vi "Disabled - Load Constants (SubVI).vi"(9 "Robot Path":string="/c/tmp/auton/", 11 "Force Reload":bool) -> (0 "Constants Numeric\nArray":dbl[](array[numeric]), 1 "error out":errorcluster, 3 "Constants Header\nArray":string[](array[string]))   [LabVIEW 2019]
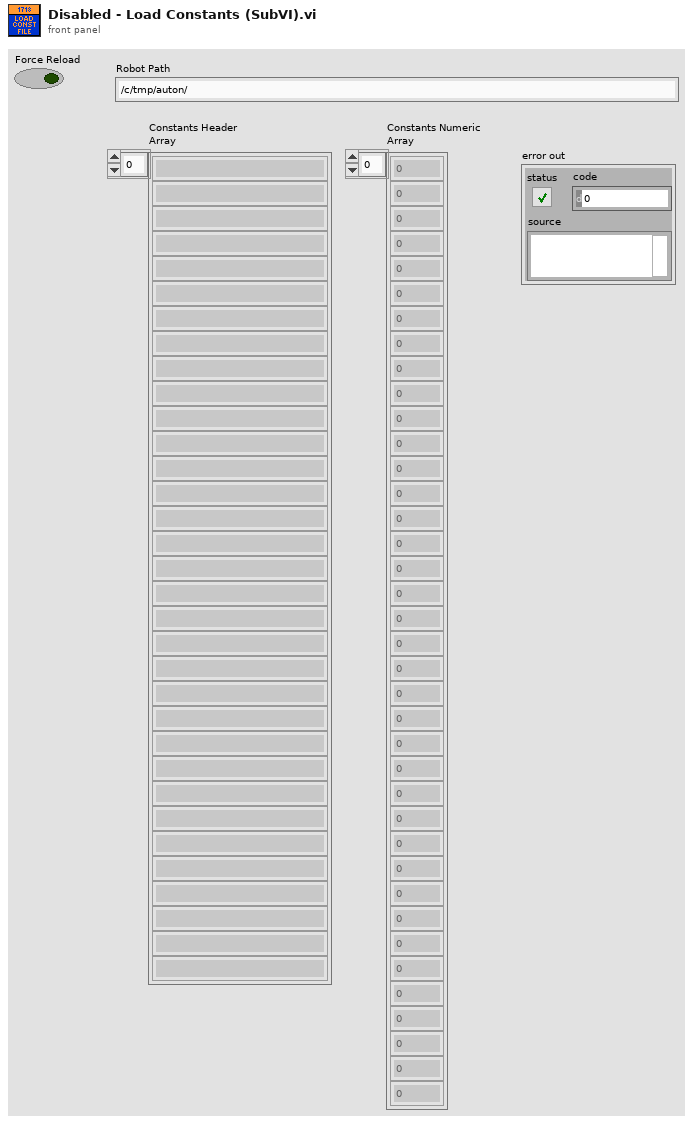
[diagram p1: front panel]
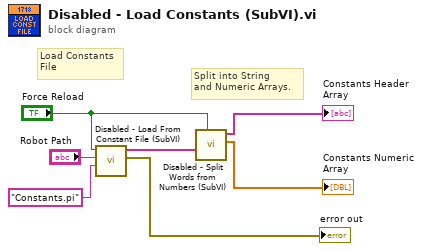
[diagram p0: block diagram]
diagram:
  # "Split into String\nand Numeric Arrays."
  # "Load Constants\nFile"
  n1 = call "Disabled - Load From Constant File (SubVI).vi"("File Name"="Constants.pi", "Robot Path"="Robot Path", "Trigger Reload"="Force Reload") -> ("error out"=→"error out":errorcluster, "Array"=w3:string[])  [unwired: 7 in]
  n2 = call "Disabled - Split Words from Numbers (SubVI).vi"("Force Reload"="Force Reload", "Input Array"=w3) -> ("Numeric Array"=→"Constants Numeric\nArray":dbl[], "Header Array"=→"Constants Header\nArray":string[])  [unwired: 8 in]
